vi "commandApplyAOSCorrectionByForces.vi"(8 "error in (no error)":errorcluster, 10 "CommandApplyAOSCorrectionByForces in":T1, 11 "Communicator in":refnum<class "Communicator.lvclass">) -> (0 "error out":errorcluster, 2 "CommandApplyAOSCorrectionByForces out":T1, 3 "Communicator out":refnum<class "Communicator.lvclass">)   [LabVIEW 2016, in "M1M3SupportCommunicator.lvlib" / "Communicator.lvclass"]
uses:
  Communicator.lvclass
  DataTypes/Topics/CommandApplyAOSCorrectionByForces.ctl
  DataTypes/Topics/Parts/CommandId.ctl
  DataTypes/Topics/M1M3SupportTopics.lvlib
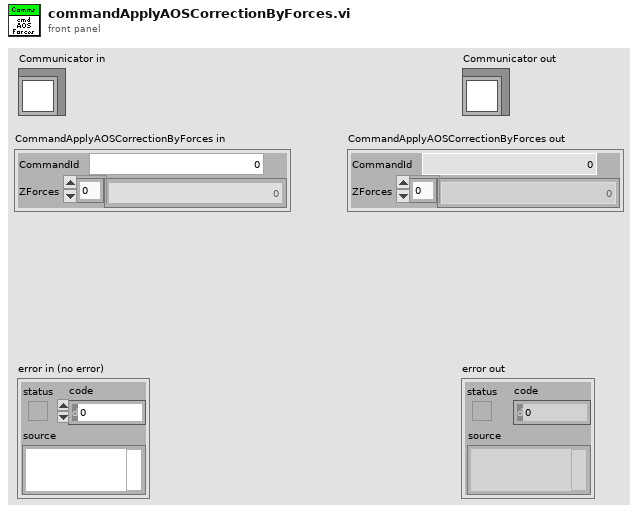
[diagram p1: front panel]
types:
  T1 = typedef "M1M3SupportTopics.lvlib/CommandApplyAOSCorrectionByForces.ctl" = cluster{"CommandId":T2, "ZForces":dbl[]}
  T2 = typedef "M1M3SupportTopics.lvlib/CommandId.ctl" = i32
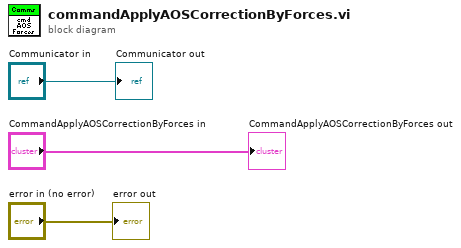
[diagram p0: block diagram]
diagram:
  "error out" <- "error in (no error)"
  "Communicator out" <- "Communicator in"
  "CommandApplyAOSCorrectionByForces out" <- "CommandApplyAOSCorrectionByForces in"
